vi "PicoScope3000aGetMaxEtsValues.vi"(8 "error in (no error)":errorcluster, 11 "handle in":i16) -> (0 "error out":errorcluster, 1 "Max etsInterleave":i16, 2 "Max etsCycles":i16, 3 "handle out":i16)   [LabVIEW 2010]
doc: "Calls GetMaxEtsValues"
uses:
  ps3000a.dll
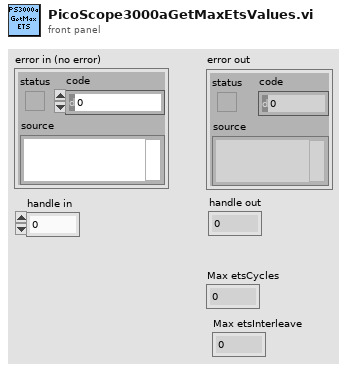
[diagram p1: front panel]
types:
  T1 = cluster{"status":bool, "code":u32, "source":string}
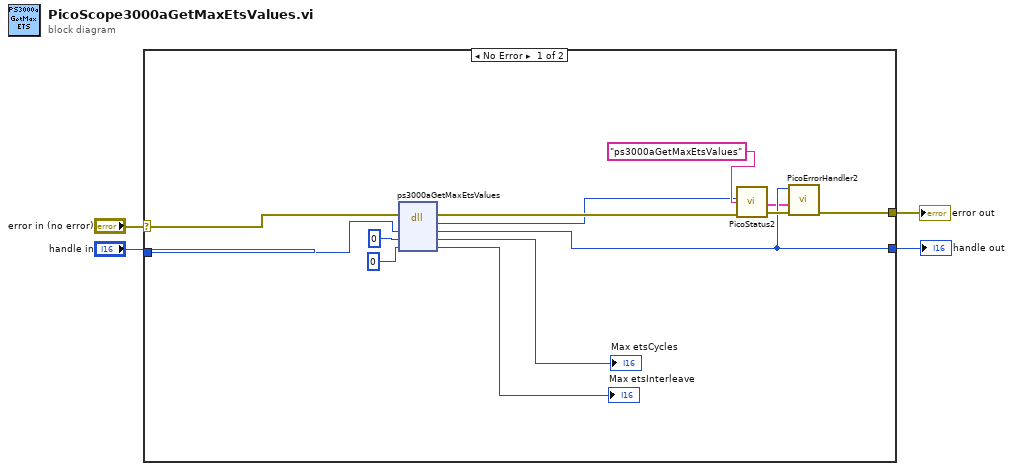
[diagram p0: block diagram]
diagram:
  n1 = case shown="No Error" "error in (no error)" {
    selector: "error in (no error)" -> [w10 w19]
    tunnel: [w16 w19] -> w2
    tunnel: "handle in" -> [w9 w18]
    tunnel: [w8 w18] -> w3
    frame No Error {
      n2 = dll-call lib="ps3000a.dll" fn="ps3000aGetMaxEtsValues" ("ps3000.dll:_ps3000_open_unit@0")(error in=w10, "handle"=w9, "etsCycles"=i16 0, "etsInterleave"=i16 0) -> (error out=w12:errorcluster, "PICO_STATUS"=w11:u32, "handle"=w8:i16, "etsCycles"=→"Max etsCycles":i16, "etsInterleave"=→"Max etsInterleave":i16)  [unwired: 2 in, 1 out]
      n3 = call "PicoStatus2.vi"("PICO source"="ps3000aGetMaxEtsValues" ("source"), "Error in"=w12, "PICO STATUS"=w11) -> ("error out"=w17:errorcluster, "PICO_STATUS out"=w5:T1)  [unwired: 5 in]
      n4 = call "PicoErrorHandler2.vi"("error in (no error)"=w17, "PICO_STATUS in"=w5, "handle In"=w8) -> ("error out"=w16:errorcluster)  [unwired: 8 in]
    }
    frame Error {
    }
  }
  "error out" <- w2
  "handle out" <- w3
